vi "MecanumCartesian.vi"(4 "Gyro Angle":dbl, 5 "X":dbl, 6 "Y":dbl, 7 "Rotation":dbl) -> (0 "Rear Right":dbl, 1 "Rear Left":dbl, 2 "Front Right":dbl, 3 "Front Left":dbl)   [LabVIEW 2013]
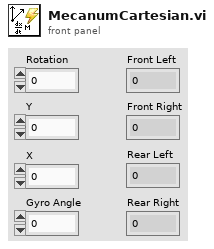
[diagram p1: front panel]
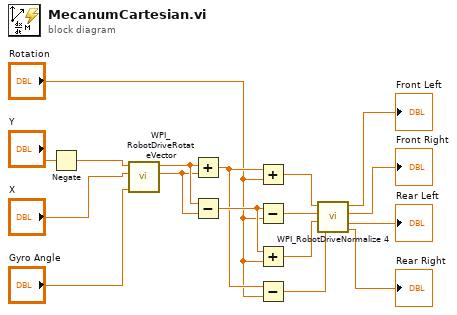
[diagram p0: block diagram]
diagram:
  n1 = Negate(x="Y") -> (-x=w16:dbl)
  n2 = call <vilib>:"WPI_RobotDriveRotateVector.vi"("Angle"="Gyro Angle", "X"="X", "Y"=w16) -> ("X'"=w12:dbl, "Y'"=w13:dbl)  [unwired: 7 out]
  n3 = Add(x=w13, y=w12) -> (x+y=w10:dbl)
  n4 = Subtract(x=w13, y=w12) -> (x-y=w11:dbl)
  n5 = Add(x=w10, y="Rotation") -> (x+y=w7:dbl)
  n6 = Subtract(x=w11, y="Rotation") -> (x-y=w8:dbl)
  n7 = Add(x=w11, y="Rotation") -> (x+y=w6:dbl)
  n8 = Subtract(x=w10, y="Rotation") -> (x-y=w5:dbl)
  n9 = call <vilib>:"WPI_RobotDriveNormalize 4.vi"("D"=w5, "C"=w6, "B"=w8, "A"=w7) -> ("D'"=→"Rear Right":dbl, "C'"=→"Rear Left":dbl, "B'"=→"Front Right":dbl, "A'"=→"Front Left":dbl)
